vi "CollectPDCAdata.vi"(11 "PDCA Collect Data In":T1) -> (3 "PDCA Data Out":string)   [LabVIEW 2011]
panel:
  out "连接的字符串":string
  out "输出簇":T1
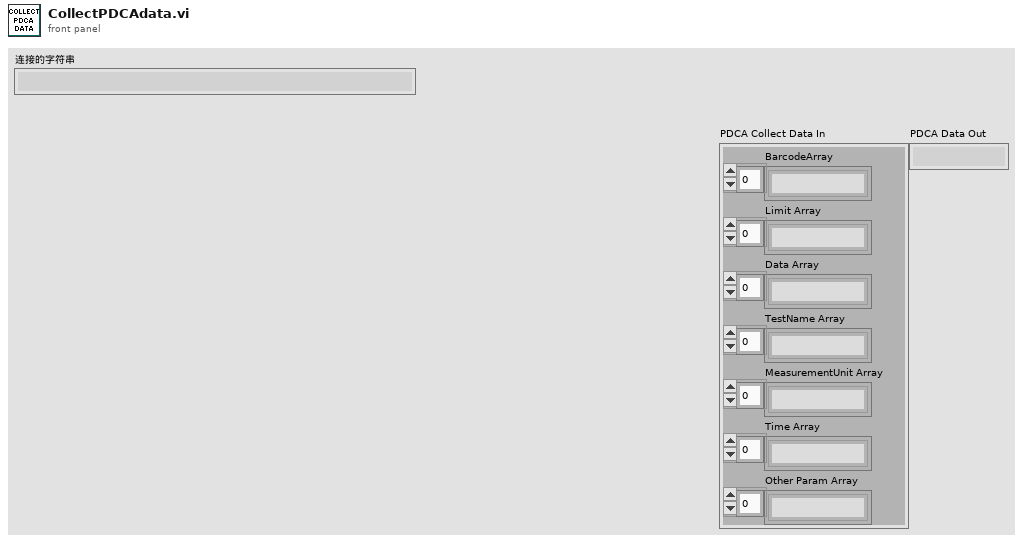
[diagram p1: front panel]
types:
  T1 = cluster{"BarcodeArray":string[], "Limit Array":string[], "Data Array":string[], "TestName Array":string[], "MeasurementUnit Array":string[], "Time Array":string[], "Other Param Array":string[]}
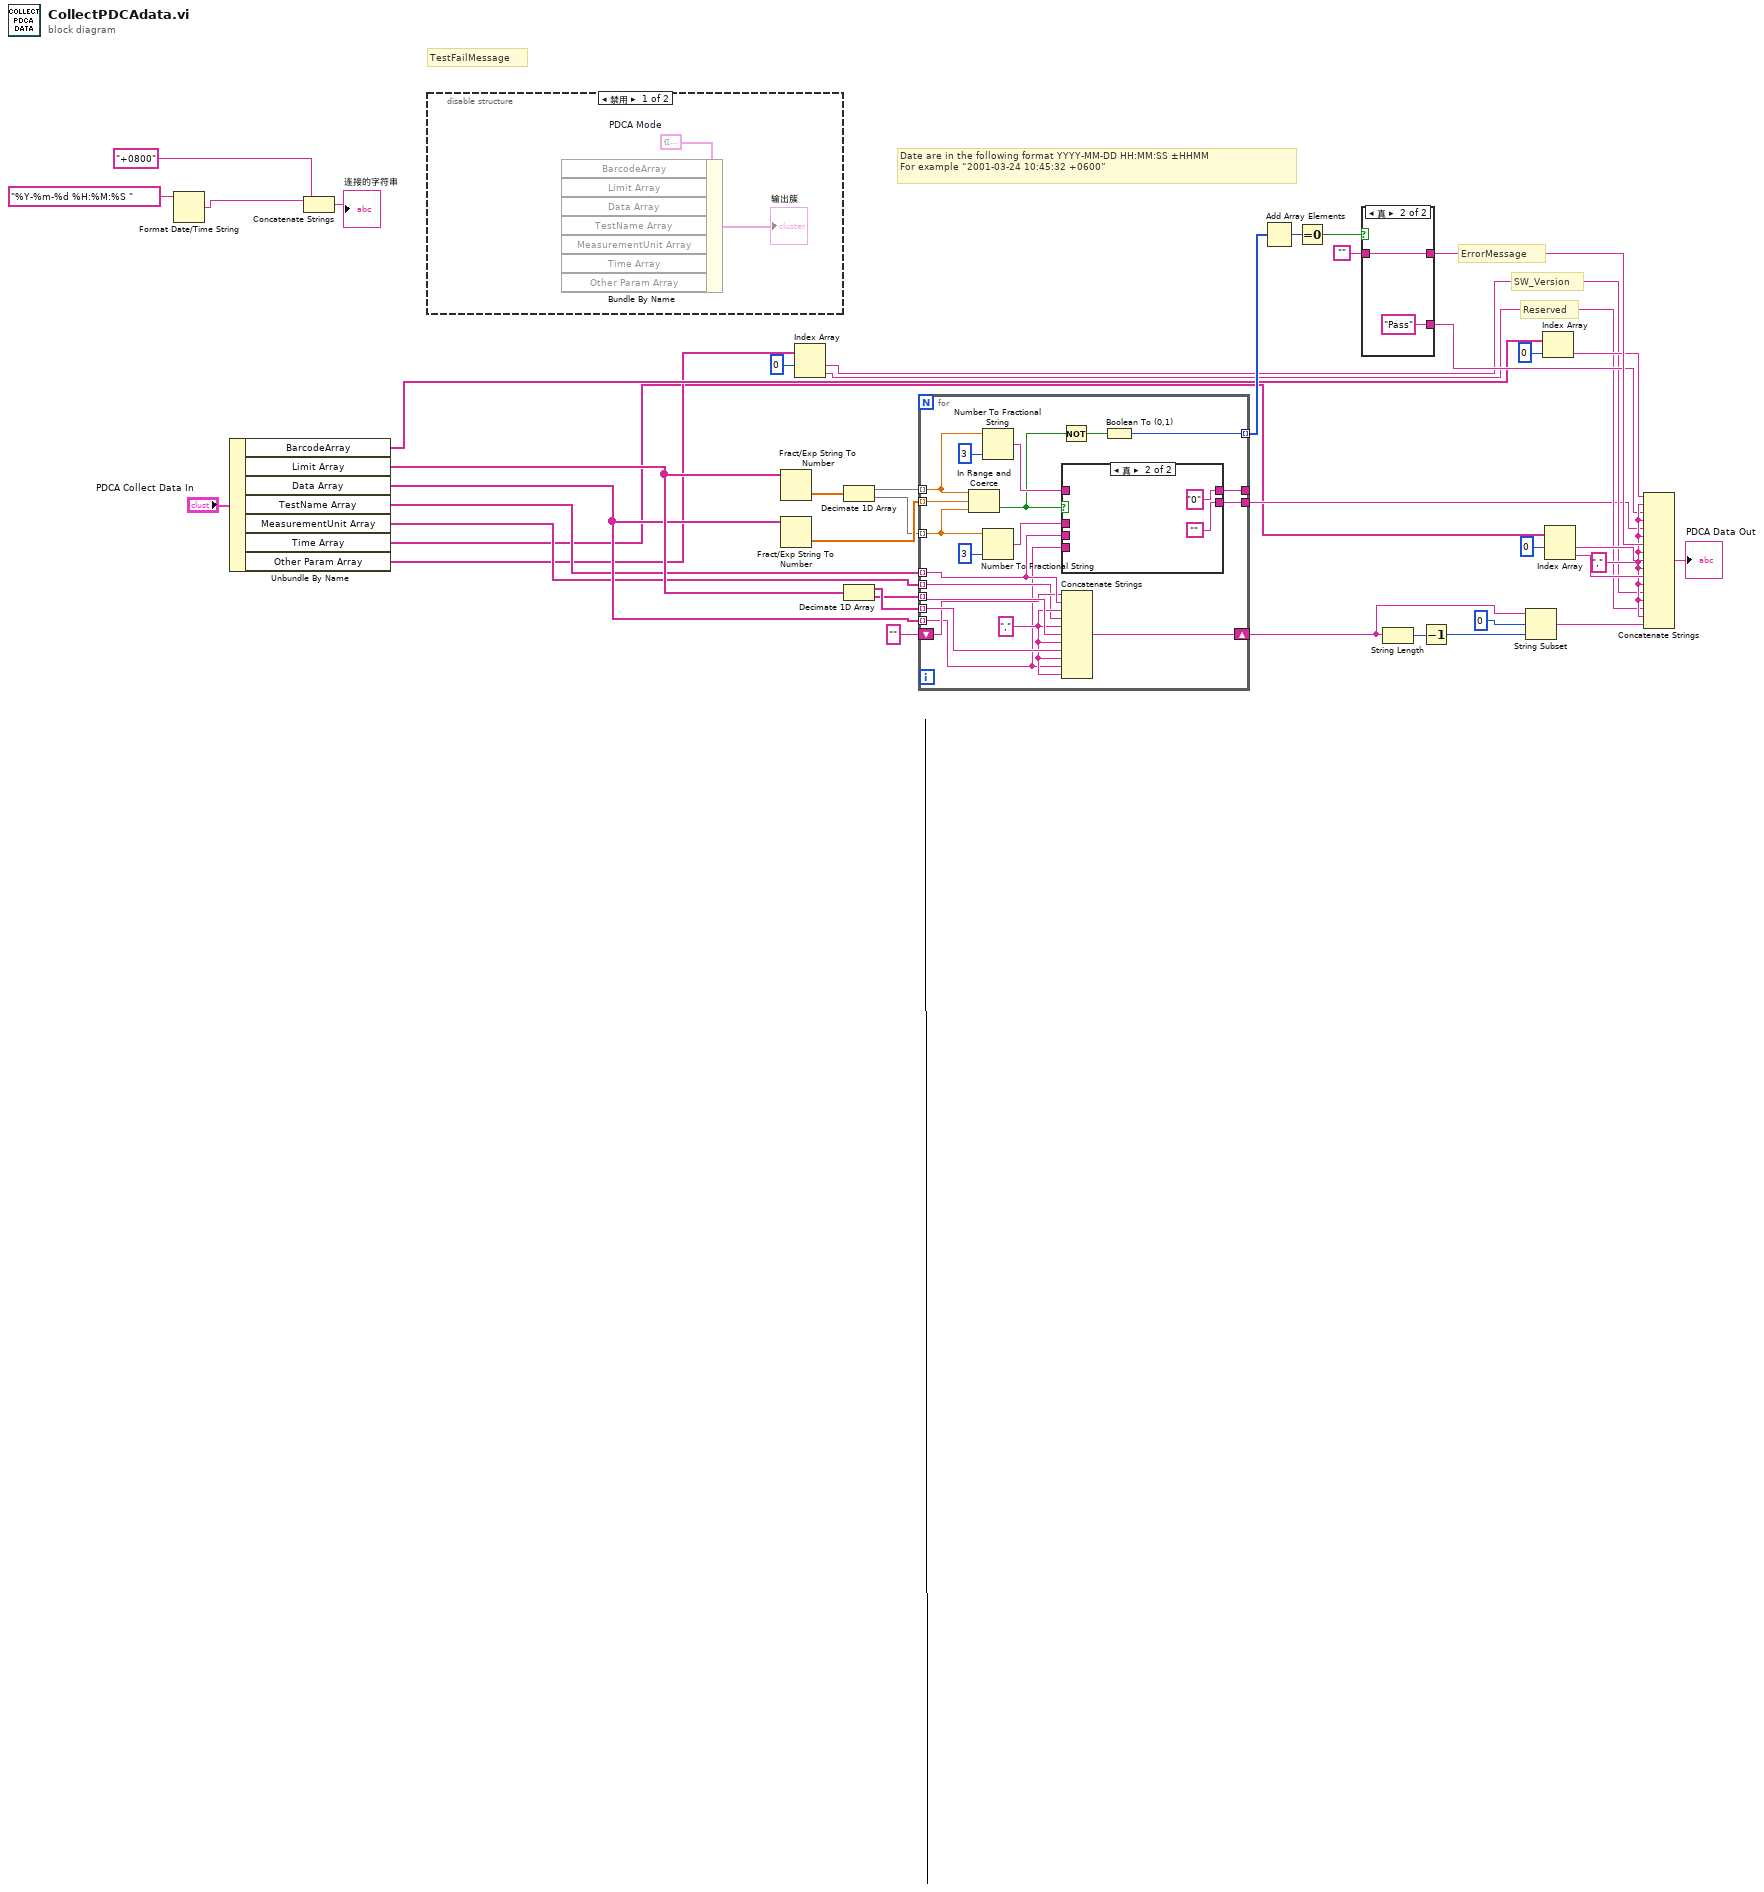
[diagram p0: block diagram]
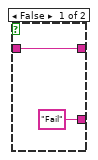
[diagram p3: hidden frame]
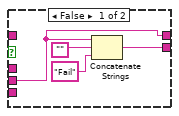
[diagram p4: hidden frame]
diagram:
  w28 = ","
  # "Date are in the following format YYYY-MM-DD HH:MM:SS ±HHMM \nFor example “2001-03-24 10:45:32 +0600”"
  # "Reserved"
  # "SW_Version"
  # "ErrorMessage"
  # "TestFailMessage"
  n1 = Format Date/Time String(time format string (%c)="%Y-%m-%d %H:%M:%S " ("时间格式字符串(%c)")) -> (date/time string=w3:string)  [unwired: 2 in]
  n2 = Unbundle By Name("PDCA Collect Data In") -> ("BarcodeArray"=w23:string[], "Limit Array"=w22:string[], "Data Array"=w21:string[], "TestName Array"=w20:string[], "MeasurementUnit Array"=w19:string[], "Time Array"=w5:string[], "Other Param Array"=w18:string[])
  n3 = Concatenate Strings(w3, "+0800" ("字符串")) -> (→"连接的字符串":string)
  n4 = disable-structure shown="禁用" {
    frame Disabled {
      w43 = T1 {"BarcodeArray"=[], "Limit Array"=[], "Data Array"=[], "TestName Array"=[], "MeasurementUnit Array"=[], "Time Array"=[], "Other Param Array"=[]}  # PDCA Mode
      n5 = Bundle By Name(cluster=w43) -> (→"输出簇":T1)  [unwired: 7 in]
    }
    frame Enabled {
    }
  }
  n6 = Fract/Exp String To Number(string=w22) -> (number=w40:dbl[])  [unwired: 3 in, 1 out]
  n7 = Fract/Exp String To Number(string=w21) -> (number=w39:dbl[])  [unwired: 3 in, 1 out]
  n8 = Index Array(array=w18, index #1=0 ("索引")) -> (element #1=w16:string, element #2=w15:string)  [unwired: 1 in]
  n9 = Decimate 1D Array(w40) -> (w38:dbl[], w37:dbl[])
  n10 = Decimate 1D Array(w22) -> (w27:string[], w26:string[])
  n11 = for {
    tunnel: w39 -> [w63] mode=indexing
    tunnel: w38 -> [w53] mode=indexing
    tunnel: w37 -> [w51] mode=indexing
    tunnel: [w62] -> w36 mode=indexing
    tunnel: w20 -> [w61] mode=indexing
    tunnel: w19 -> [w55] mode=indexing
    tunnel: w27 -> [w59] mode=indexing
    tunnel: w26 -> [w60] mode=indexing
    tunnel: w21 -> [w54] mode=indexing
    shift-right: [w56] -> w9
    shift-left: "" -> [w57]
    tunnel: [w47] -> _
    tunnel: [w44] -> w14
    w58 = "," ("字符串")
    n12 = In Range and Coerce(upper limit=w53, x=w63, lower limit=w51) -> (In Range?=w46:bool)  [unwired: 1 out]
    n13 = Number To Fractional String(number=w53, precision (6)=i16 3 ("精度(6)")) -> (F-format string=w49:string)  [unwired: 2 in]
    n14 = Number To Fractional String(number=w51, precision (6)=i16 3 ("精度(6)")) -> (F-format string=w48:string)  [unwired: 2 in]
    n15 = Not(x=w46) -> (.not. x?=w45:bool)
    n16 = case shown="真" w46 {
      tunnel: w61 -> [w67 _]
      tunnel: [w64 ""] -> w44
      tunnel: w54 -> [_ _]
      tunnel: w49 -> [_ _]
      tunnel: w48 -> [_ _]
      tunnel: [w67 "0" ("字符串")] -> w47
      frame False {
        n17 = Concatenate Strings(w67, "", "Fail" ("字符串")) -> (w64:string)
      }
      frame True {
      }
    }
    n18 = Concatenate Strings(w57, w61, w58, w55, w58, w60, w58, w59, w58, w54, w58) -> (w56:string)
    n19 = Boolean To (0,1)(Boolean=w45) -> (0, 1=w62:i16)
  }
  n20 = Add Array Elements(numeric array=w36) -> (sum=w35:i16)
  n21 = Equal To 0?(x=w35) -> (x = 0?=w34:bool)
  n22 = case shown="真" w34 {
    tunnel: ["Fail" "Pass"] -> w24
    tunnel: [w70 w72] -> w32
    tunnel: "" -> [w70 w72]
    frame False {
    }
    frame True {
    }
  }
  n23 = String Length(string=w9) -> (length=w11:i32)
  n24 = Decrement(x=w11) -> (x-1=w10:i32)
  n25 = String Subset(string=w9, offset (0)=0 ("偏移量(0)"), length (rest)=w10) -> (substring=w7:string)
  n26 = Index Array(array=w23, index=0 ("索引")) -> (element=w25:string)
  n27 = Index Array(array=w5, index #1=0 ("索引")) -> (element #1=w30:string, element #2=w29:string)  [unwired: 1 in]
  n28 = Concatenate Strings(w25, w28, w24, w28, w14, w28, w32, w28, w30, w28, w29, w28, w16, w28, w15, w28, w7) -> (→"PDCA Data Out":string)
